vi "Check Serial data.vi"(8 "error in":errorcluster, 11 "Buffer in":string) -> (0 "error IO":errorcluster, 3 "Good?":bool)   [LabVIEW 2019]
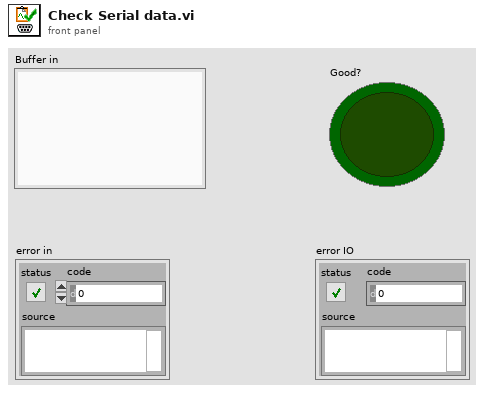
[diagram p1: front panel]
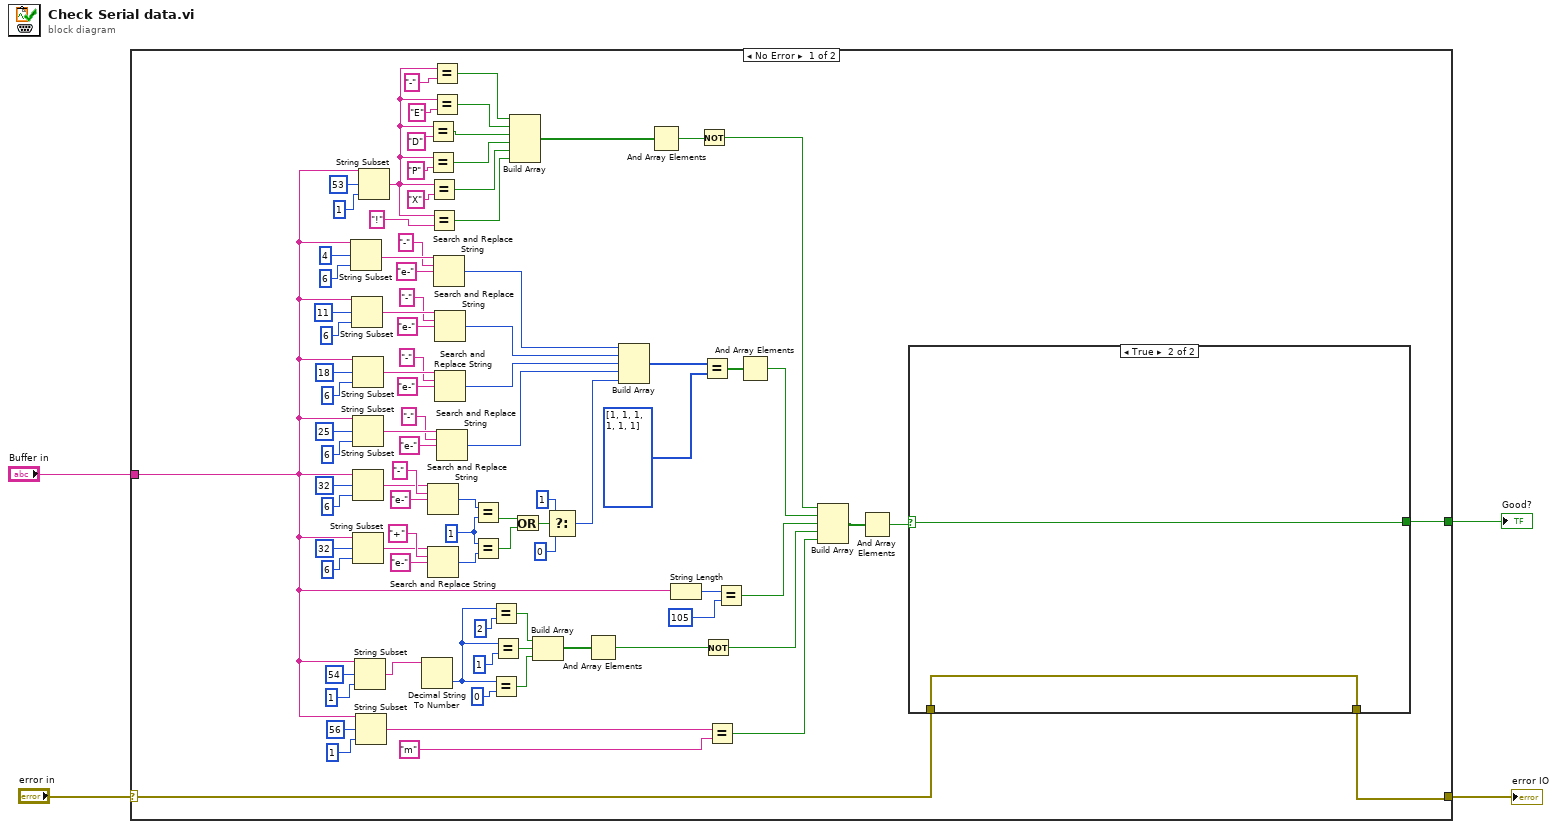
[diagram p0: block diagram]
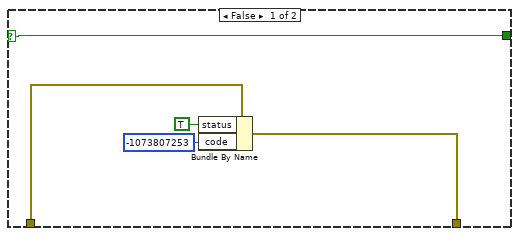
[diagram p2: hidden frame]
diagram:
  n1 = case shown="No Error" "error in" {
    selector: "error in" -> [w23 w104]
    tunnel: "Buffer in" -> [w11 _]
    tunnel: [w24 w104] -> w2
    tunnel: [w22 _] -> w1
    frame No Error {
      w9 = 1
      n2 = String Subset(string=w11, offset (0)=4, length (rest)=6 ("length (rest)")) -> (substring=w87:string)
      n3 = String Subset(string=w11, offset (0)=11, length (rest)=6 ("length (rest)")) -> (substring=w90:string)
      n4 = String Subset(string=w11, offset (0)=18, length (rest)=6 ("length (rest)")) -> (substring=w93:string)
      n5 = String Subset(string=w11, offset (0)=25, length (rest)=6 ("length (rest)")) -> (substring=w96:string)
      n6 = String Subset(string=w11, offset (0)=32, length (rest)=6 ("length (rest)")) -> (substring=w82:string)
      n7 = String Subset(string=w11, offset (0)=32, length (rest)=6 ("length (rest)")) -> (substring=w14:string)
      n8 = String Subset(string=w11, offset (0)=54, length (rest)=1 ("length (rest)")) -> (substring=w81:string)
      n9 = String Subset(string=w11, offset (0)=56, length (rest)=1 ("length (rest)")) -> (substring=w55:string)
      n10 = String Subset(string=w11, offset (0)=53, length (rest)=1 ("length (rest)")) -> (substring=w44:string)
      n11 = Decimal String To Number(string=w81) -> (number=w53:i32)  [unwired: 2 in, 1 out]
      n12 = Equal?(x=w44, y="D") -> (x = y?=w35:bool)
      n13 = Equal?(x=w44, y="P") -> (x = y?=w34:bool)
      n14 = Search and Replace String(input string=w82, search string="-", replace string="e-" ("replace string (\"\")")) -> (number of replacements=w8:i32)  [unwired: 5 in, 3 out]
      n15 = Search and Replace String(input string=w14, search string="+", replace string="e-" ("replace string (\"\")")) -> (number of replacements=w7:i32)  [unwired: 5 in, 3 out]
      n16 = Equal?(x=w44, y="X") -> (x = y?=w33:bool)
      n17 = Equal?(x=w44, y="!") -> (x = y?=w32:bool)
      n18 = Equal?(x=w44, y="-") -> (x = y?=w37:bool)
      n19 = Equal?(x=w44, y="E") -> (x = y?=w36:bool)
      n20 = Search and Replace String(input string=w87, search string="-", replace string="e-" ("replace string (\"\")")) -> (number of replacements=w64:i32)  [unwired: 5 in, 3 out]
      n21 = Search and Replace String(input string=w90, search string="-", replace string="e-" ("replace string (\"\")")) -> (number of replacements=w61:i32)  [unwired: 5 in, 3 out]
      n22 = Search and Replace String(input string=w93, search string="-", replace string="e-" ("replace string (\"\")")) -> (number of replacements=w62:i32)  [unwired: 5 in, 3 out]
      n23 = Search and Replace String(input string=w96, search string="-", replace string="e-" ("replace string (\"\")")) -> (number of replacements=w63:i32)  [unwired: 5 in, 3 out]
      n24 = Equal?(x=w8, y=w9) -> (x = y?=w6:bool)
      n25 = Equal?(x=w9, y=w7) -> (x = y?=w5:bool)
      n26 = Equal?(x=w53, y=2) -> (x = y?=w47:bool)
      n27 = Equal?(x=w53, y=0) -> (x = y?=w49:bool)
      n28 = Equal?(x=w53, y=1) -> (x = y?=w48:bool)
      n29 = Build Array(w37, w36, w35, w34, w33, w32) -> (w31:bool[])
      n30 = Or(x=w6, y=w5) -> (x .or. y?=w10:bool)
      n31 = Build Array(w47, w48, w49) -> (w46:bool[])
      n32 = Select(t=1, s=w10, f=0) -> (s? t:f=w18:i32)
      n33 = And Array Elements(Boolean array=w46) -> (logical AND=w45:bool)
      n34 = Build Array(w64, w61, w62, w63, w18) -> (w60:i32[])
      n35 = And Array Elements(Boolean array=w31) -> (logical AND=w21:bool)
      n36 = String Length(string=w11) -> (length=w57:i32)
      n37 = Not(x=w21) -> (.not. x?=w20:bool)
      n38 = Equal?(x=w60, y=i32[] [1, 1, 1, 1, 1, 1]) -> (x = y?=w59:bool[])
      n39 = Not(x=w45) -> (.not. x?=w30:bool)
      n40 = Equal?(x=w55, y="m") -> (x = y?=w29:bool)
      n41 = Equal?(x=w57, y=105) -> (x = y?=w28:bool)
      n42 = And Array Elements(Boolean array=w59) -> (logical AND=w27:bool)
      n43 = Build Array(w20, w27, w28, w30, w29) -> (w26:bool[])
      n44 = And Array Elements(Boolean array=w26) -> (logical AND=w25:bool)
      n45 = case shown="True" w25 {
        selector: w25 -> [w98 w102]
        tunnel: [w100 w103] -> w24
        tunnel: w23 -> [w101 w103]
        tunnel: [w98 w102] -> w22
        frame False {
          n46 = Bundle By Name(cluster=w101, "status"=TRUE, "code"=-1073807253 ("specific error code to clear (0: all)")) -> (w100:errorcluster)
        }
        frame True {
        }
      }
    }
    frame Error {
    }
  }
  "error IO" <- w2
  "Good?" <- w1
